vi "Reinitialize All.vi"(8 "error in (no error)":errorcluster, 11 "Hot And Cold Source Unit Model in":refnum<class "Hot And Cold Source Unit Model.lvclass">) -> (0 "error out":errorcluster, 3 "Hot And Cold Source Unit Model out":refnum<class "Hot And Cold Source Unit Model.lvclass">)   [LabVIEW 2013, in "Hot And Cold Source Unit Model.lvlib" / "Hot And Cold Source Unit Model.lvclass"]
uses:
  Hot And Cold Source Unit Model.lvclass
  Hot And Cold Source Unit Model.lvclass/Hot And Cold Source Unit Model.ctl
  <vilib>/ActorFrameworkMVC/View Observer/View Registry/View Registry.lvclass/View Registry.ctl
  Hot And Cold Source Unit Model Messages/Abstract Initialize Hot And Cold Source Unit Msg/Abstract Initialize Hot And Cold Source Unit Msg.lvclass
  <vilib>/ActorFrameworkMVC/View Observer/Data Message/Data Message.lvclass
  <vilib>/ActorFrameworkMVC/View Observer/View Registry/View Registry.lvclass
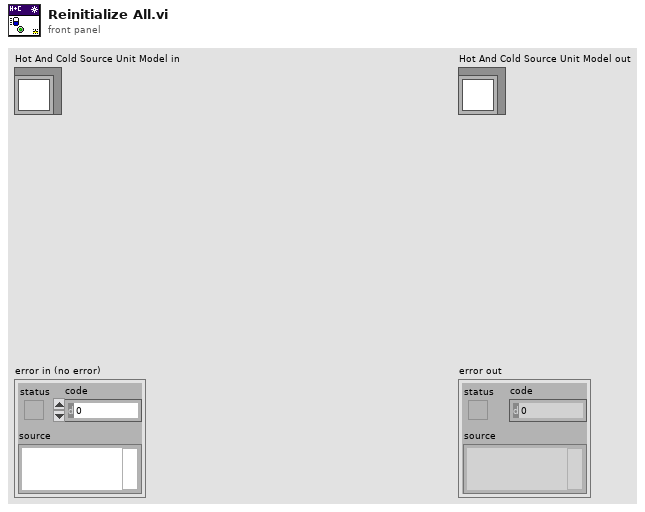
[diagram p1: front panel]
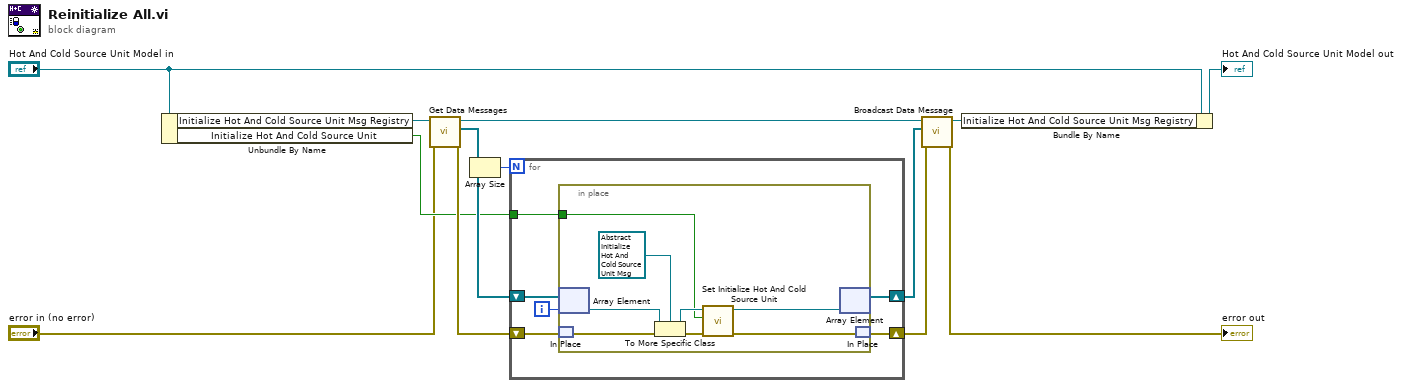
[diagram p0: block diagram]
diagram:
  n1 = Unbundle By Name("Hot And Cold Source Unit Model in") -> ("Initialize Hot And Cold Source Unit Msg Registry"=w13:refnum<class "View Registry.lvclass">, "Initialize Hot And Cold Source Unit"=w8:bool)
  n2 = call <vilib>:"Get Data Messages.vi"("error in (no error)"="error in (no error)", "View Registry in"=w13) -> ("error out"=w9:errorcluster, "Data Messages"=w10:refnum<class "Data Message.lvclass">[], "View Registry out"=w12:refnum<class "View Registry.lvclass">)  [unwired: 7 in]
  n3 = Array Size(array=w10) -> (size(s)=w11:i32)
  n4 = for {
    N: w11 -> [_]
    shift-right: [w18] -> w7
    shift-left: w10 -> [w19]
    shift-right: [w15] -> w6
    shift-left: w9 -> [w17]
    tunnel: w8 -> [w16]
    i -> [w14]
    n5 = in-place {
      in-place-border: w16 -> [w20]
      n6 = in-place-array #1(w19, w14) -> (w25:refnum<class "Data Message.lvclass">)
      n7 = in-place-match #2(w17) -> (w27:errorcluster)
      n8 = To More Specific Class(target class=refnum<class "Abstract Initialize Hot And Cold Source Unit Msg.lvclass"> refnum ("Hot And Cold Source Unit Model.lvlib:Abstract Initialize Hot And Cold Source Unit Msg.lvclass"), reference=w25, error in=w27) -> (specific class reference=w21:refnum<class "Abstract Initialize Hot And Cold Source Unit Msg.lvclass">, error out=w24:errorcluster)
      n9 = call "Set Initialize Hot And Cold Source Unit.vi"("error in (no error)"=w24, "Initialize Hot And Cold Source Unit"=w20, "Abstract Initialize Hot And Cold Source Unit Msg in"=w21) -> ("error out"=w23:errorcluster, "Abstract Initialize Hot And Cold Source Unit Msg out"=w22:refnum<class "Abstract Initialize Hot And Cold Source Unit Msg.lvclass">)  [unwired: 7 in]
      n10 = in-place-array #1(w22) -> (w18:refnum<class "Data Message.lvclass">[])  [unwired: 1 out]
      n11 = in-place-match #2(w23) -> (w15:errorcluster)
    }
  }
  n12 = call <vilib>:"Broadcast Data Message.vi"("error in (no error)"=w6, "Data Messages"=w7, "View Registry in"=w12) -> ("error out"=→"error out":errorcluster, "View Registry out"=w5:refnum<class "View Registry.lvclass">)  [unwired: 7 in]
  n13 = Bundle By Name(cluster="Hot And Cold Source Unit Model in", "Initialize Hot And Cold Source Unit Msg Registry"=w5) -> (→"Hot And Cold Source Unit Model out":refnum<class "Hot And Cold Source Unit Model.lvclass">)
